vi "assert_cancel_token.vi"(8 "error in (no error)":errorcluster, 10 "abort_in":bool) -> (0 "error out":errorcluster, 2 "abort_out":bool)   [LabVIEW 2021, in "system.threading.lvclass"]
uses:
  system.threading.lvclass
  system.threading.lvclass/system.threading.ctl
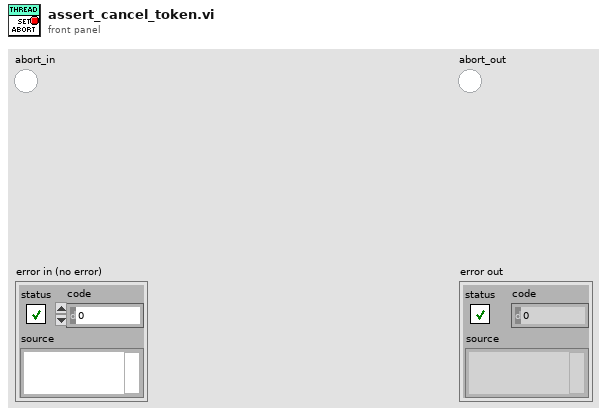
[diagram p1: front panel]
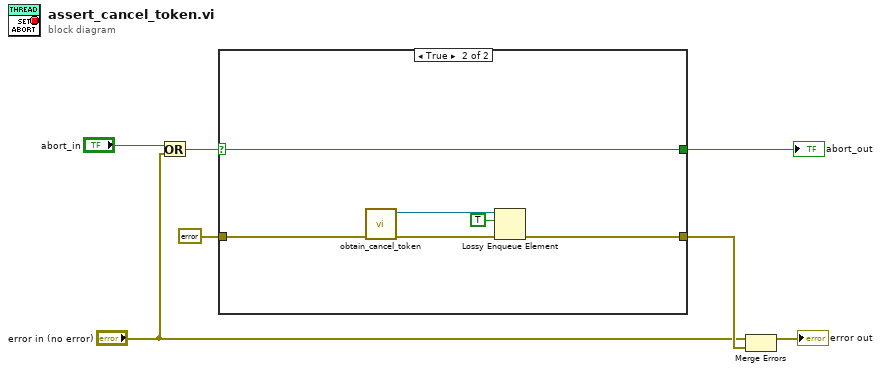
[diagram p0: block diagram]
diagram:
  n1 = Or(x="abort_in", y="error in (no error)") -> (x .or. y?=w6:bool)
  n2 = case shown="True" w6 {
    selector: w6 -> [w9 w12]
    tunnel: [w9 w12] -> w5
    tunnel: errorcluster {"status"=FALSE, "code"=0, "source"=""} ("error in (no error)") -> [w8 w11]
    tunnel: [w8 w10] -> w2
    frame False {
    }
    frame True {
      n3 = call "obtain_cancel_token.vi"("error in (no error)"=w11) -> ("error out"=w15:errorcluster, "cancel_token"=w14:refnum<queue>)  [unwired: 9 in]
      n4 = Lossy Enqueue Element(queue=w14, element=TRUE, error in (no error)=w15) -> (error out=w10:errorcluster)  [unwired: 3 out]
    }
  }
  "abort_out" <- w5
  n5 = Merge Errors("error in (no error)", w2) -> (→"error out":errorcluster)
